vi "Read Loop Times.vi"(0 "FPGA API in":refnum<class "FPGA API.lvclass">, 11 "error in (no error)":errorcluster) -> (4 "FPGA API out":refnum<class "FPGA API.lvclass">, 6 "dt(tiks) AI loop":u32, 8 "dt(tiks) DI loop":u32, 10 "dt(tiks) DO loop":u32, 14 "dt (ticks) AO Loop":u32, 15 "error out":errorcluster)   [LabVIEW 2019, in "FPGA API.lvclass"]
uses:
  FPGA API.lvclass
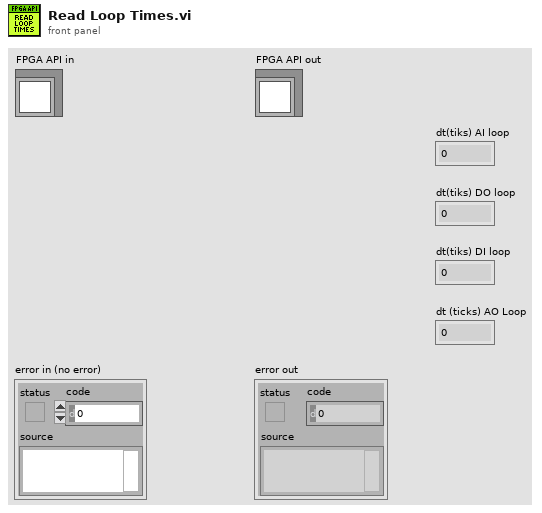
[diagram p1: front panel]
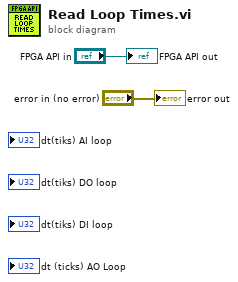
[diagram p0: block diagram]
diagram:
  "error out" <- "error in (no error)"
  "FPGA API out" <- "FPGA API in"
